vi "MemFromHTML_+CreatedTempPath_xSWF.vi"(6 "Identifying_String":string="img src=\"", 7 "user event in":refnum<user-event>, 8 "error in (no error)":errorcluster, 9 "Dencrypted text":string, 10 "FolderName":string, 11 "Folder_Mgmt":refnum<class "Folder_Mgmt.lvclass">) -> (0 "error out":errorcluster, 1 "ModifyedHTML":string, 2 "TemporaryFiles":path[](array[path]), 3 "Folder_Mgmt 2":refnum<class "Folder_Mgmt.lvclass">)   [LabVIEW 2016, in "Folder_Mgmt.lvclass"]
uses:
  Folder_Mgmt.lvclass
  Folder_Mgmt.lvclass/Folder_Mgmt.ctl
panel:
  out "before substring":string
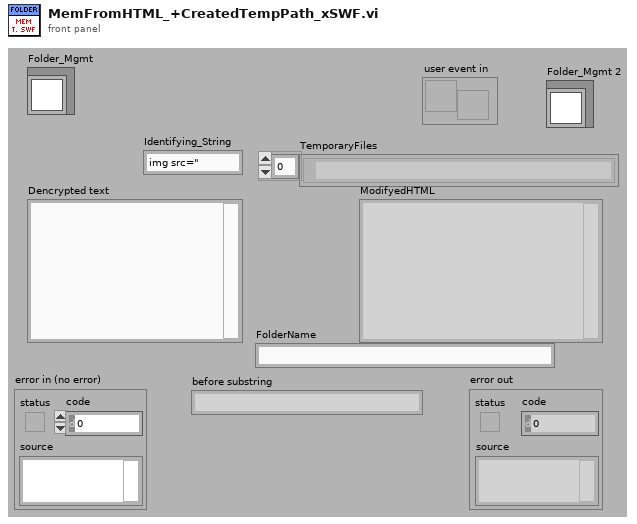
[diagram p1: front panel]
types:
  T1 = cluster{"Timeout":i32, "WaitPlease":bool, "StopWait":bool}
  T2 = enum16{"open", "replace", "create", "open or create", "replace or create", "replace or create with confirmation"}
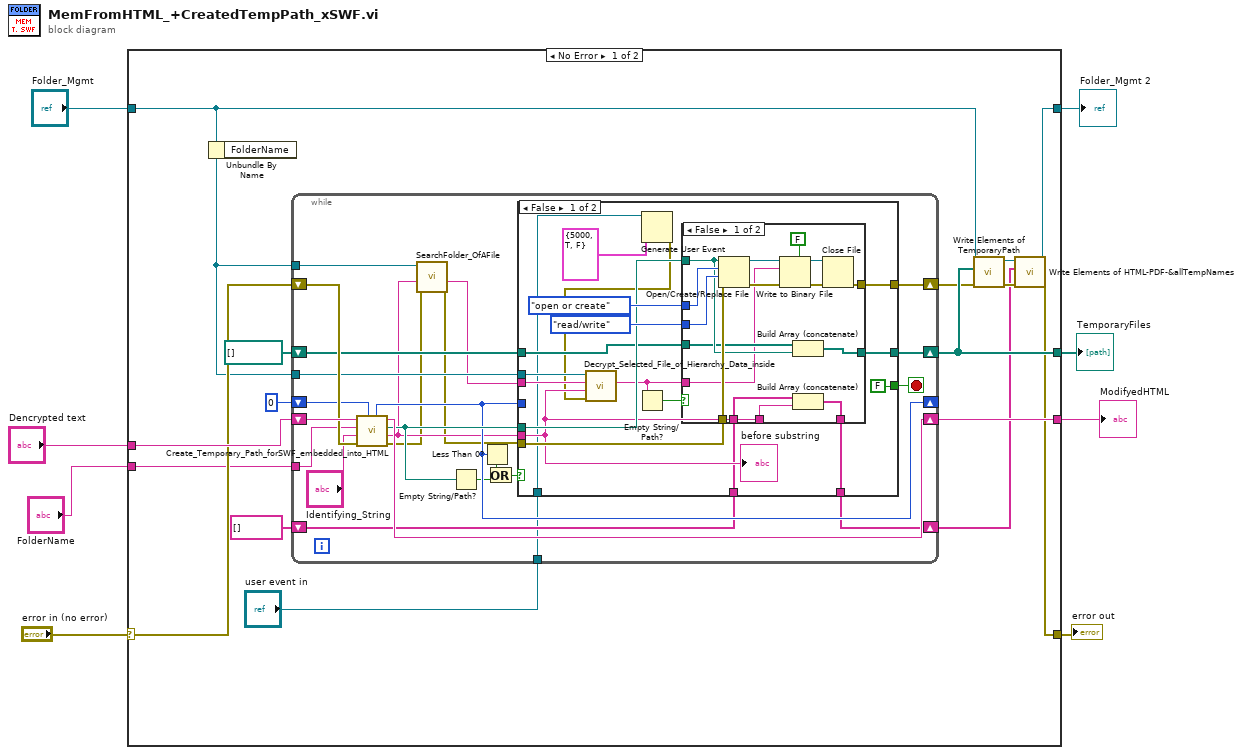
[diagram p0: block diagram]
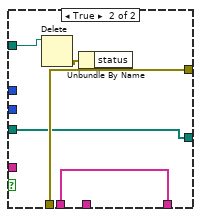
[diagram p2: hidden frame]
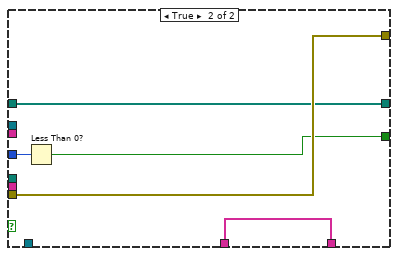
[diagram p3: hidden frame]
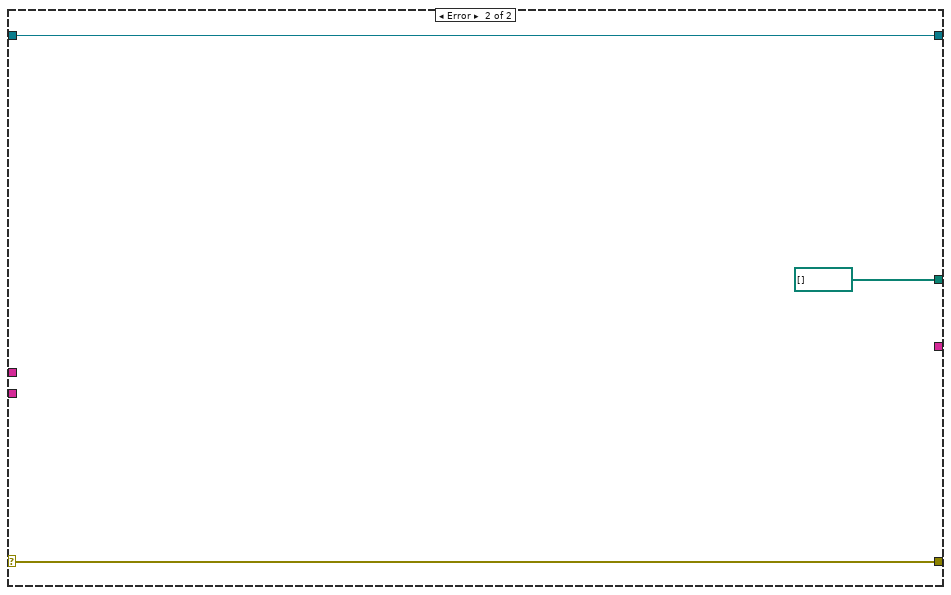
[diagram p4: hidden frame]
diagram:
  n1 = case shown="No Error" "error in (no error)" {
    selector: "error in (no error)" -> [w22 w95]
    tunnel: [w14 w95] -> w7
    tunnel: [w12 w94] -> w3
    tunnel: "Folder_Mgmt" -> [w11 w94]
    tunnel: "Dencrypted text" -> [w23 _]
    tunnel: [w19 path[] []] -> w5
    tunnel: [w21 _] -> w4
    tunnel: "FolderName" -> [w10 _]
    frame No Error {
      n2 = Unbundle By Name(w11) -> ()  [unwired: 1 out]
      n3 = while {
        tunnel: w11 -> [w44]
        shift-right: [w48] -> w18
        shift-left: w22 -> [w45]
        shift-right: [w46] -> w21
        shift-left: w23 -> [w47]
        shift-right: [w38] -> _
        shift-left: 0 ("offset past match") -> [w40]
        shift-right: [w42] -> w19
        shift-left: path[] [] -> [w35]
        shift-right: [w32] -> w15
        shift-left: string[] [] -> [w33]
        tunnel: w11 -> [w31]
        tunnel: w10 -> [w26]
        tunnel: "user event in" -> [w25]
        stop <- w41 stop-if-true
        n4 = call "Create_Temporary_Path_forSWF_embedded_into_HTML.vi"("offset past match"=w40, "error in (no error)"=w45, "Identifying_String"="Identifying_String", "FolderName"=w26, "Dencrypted text"=w47) -> ("error out"=w29:errorcluster, "fileName"=w30:string, "Temp_PATH"=w43:path, "HTML_wPathChanged"=w46:string, "offset past match"=w38:i32)  [unwired: 2 in]
        n5 = call "SearchFolder_OfAFile.vi"("Folder_Mgmt out"=w31, "FileToSearch"=w30, "error in (no error)"=w29) -> ("FolderOfFile"=w27:string, "error out"=w28:errorcluster)  [unwired: 5 in, 1 out]
        n6 = Empty String/Path?(string/path=w43) -> (empty?=w34:bool)
        n7 = Less Than 0?(x=w38) -> (x < 0?=w37:bool)
        n8 = Or(x=w37, y=w34) -> (x .or. y?=w39:bool)
        n9 = case shown="False" w39 {
          tunnel: [w64 w92] -> w48
          tunnel: w30 -> [w54 _]
          tunnel: w28 -> [w63 w92]
          tunnel: w44 -> [w62 _]
          tunnel: w27 -> [w61 _]
          tunnel: w43 -> [w60 _]
          tunnel: [w58 w91] -> w42
          tunnel: [FALSE w88] -> w41
          tunnel: w38 -> [_ w89]
          tunnel: w35 -> [w57 w91]
          tunnel: w33 -> [w53 w90]
          tunnel: [w52 w90] -> w32
          tunnel: w25 -> [w51 _]
          frame False {
            n10 = Generate User Event(user event=w51, event data cluster=T1 {"Timeout"=5000, "WaitPlease"=TRUE, "StopWait"=FALSE} ("event data")) -> (error out=w49:errorcluster)  [unwired: 2 in, 1 out]
            n11 = call-dynamic "Decrypt_Selected_File_of_Hierarchy_Data_inside.vi"("error in (no error)"=w49, "FileName"=w54, "SubFolderName"=w61, "object in"=w62) -> ("Dencrypted text"=w56:string)  [unwired: 4 in, 3 out]
            n12 = Empty String/Path?(string/path=w56) -> (empty?=w55:bool)
            n13 = case shown="False" w55 {
              tunnel: enum16{"read/write", "read-only", "write-only"}."read/write" ("access (0:read/write)") -> [w78 _]
              tunnel: T2."open or create" ("operation (0:open)") -> [w77 _]
              tunnel: [w75 w87] -> w64
              tunnel: w63 -> [w74 w87]
              tunnel: w60 -> [w73 w85]
              tunnel: [w72 w86] -> w58
              tunnel: w57 -> [w71 w86]
              tunnel: w56 -> [w70 _]
              tunnel: w54 -> [w69 _]
              tunnel: w53 -> [w68 w83]
              tunnel: [w67 w83] -> w52
              frame False {
                n14 = Open/Create/Replace File(file path (use dialog)=w73, error in=w74, operation (0:open)=w77, access (0:read/write)=w78) -> (refnum out=w79:refnum<file>, error out=w80:errorcluster)  [unwired: 2 in, 1 out]
                n15 = Write to Binary File(file (use dialog)=w79, data=w70, error in=w80, 5:FALSE ("prepend array or string size? (T)")) -> (refnum out=w82:refnum<file>, error out=w81:errorcluster)  [unwired: 2 in, 1 out]
                n16 = Build Array (concatenate)(w71, w73) -> (w72:path[])
                n17 = Build Array (concatenate)(w68, w69) -> (w67:string[])
                n18 = Close File(refnum=w82, error in=w81) -> (error out=w75:errorcluster)  [unwired: 1 out]
              }
              frame True {
                n19 = Delete(path (use dialog)=w85) -> (error out=w84:errorcluster)  [unwired: 4 in, 2 out]
                n20 = Unbundle By Name(w84) -> ()  [unwired: 1 out]
              }
            }
            "before substring" <- w54
          }
          frame True {
            n21 = Less Than 0?(x=w89) -> (x < 0?=w88:bool)
          }
        }
      }
      n22 = call "Write Elements of TemporaryPath.vi"("error in (no error)"=w18, "Paths"=w19, "Folder_Mgmt"=w11) -> ("error out"=w16:errorcluster, "Folder_Mgmt 2"=w13:refnum<class "Folder_Mgmt.lvclass">)  [unwired: 7 in]
      n23 = call "Write Elements of HTML-PDF-&allTempNames.vi"("error in (no error)"=w16, "Array"=w15, "Folder_Mgmt"=w13) -> ("error out"=w14:errorcluster, "Folder_Mgmt 2"=w12:refnum<class "Folder_Mgmt.lvclass">)  [unwired: 7 in]
    }
    frame Error {
    }
  }
  "error out" <- w7
  "TemporaryFiles" <- w5
  "ModifyedHTML" <- w4
  "Folder_Mgmt 2" <- w3
